vi "折叠行_symbols.vi"(8 "错误输入（无错误）":errorcluster, 11 "引用":refnum<k24>) -> (0 "错误输出":errorcluster, 3 "引用输出":refnum<k24>)   [LabVIEW 2018]
uses:
  ScintillaNET.dll
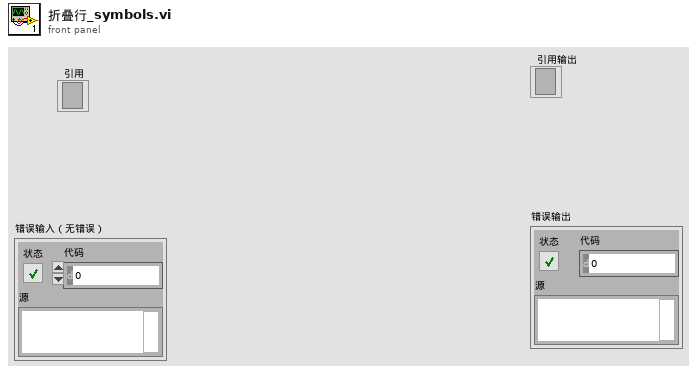
[diagram p1: front panel]
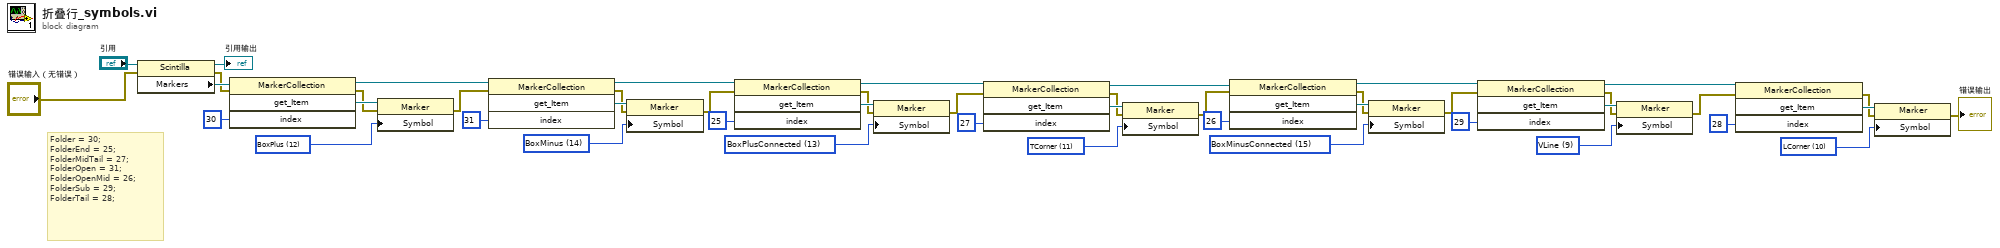
[diagram p0: block diagram]
diagram:
  w20 = 10 items=["Circle"=0, "RoundRect"=1, "Arrow"=2, "SmallRect"=3, "ShortArrow"=4, "Empty"=5, "ArrowDown"=6, "Minus"=7, "Plus"=8, "VLine"=9, "LCorner"=10, "TCorner"=11, "BoxPlus"=12, "BoxPlusConnected"=13, "BoxMinus"=14, "BoxMinusConnected"=15, "LCornerCurve"=16, "TCornerCurve"=17, "CirclePlus"=18, "CirclePlusConnected"=19, "CircleMinus"=20, "CircleMinusConnected"=21, "Background"=22, "DotDotDot"=23, "Arrows"=24, "FullRect"=26, "LeftRect"=27, "Available"=28, "Underline"=29, "RgbaImage"=30, "Bookmark"=31] ("Symbol")
  w22 = 9 items=["Circle"=0, "RoundRect"=1, "Arrow"=2, "SmallRect"=3, "ShortArrow"=4, "Empty"=5, "ArrowDown"=6, "Minus"=7, "Plus"=8, "VLine"=9, "LCorner"=10, "TCorner"=11, "BoxPlus"=12, "BoxPlusConnected"=13, "BoxMinus"=14, "BoxMinusConnected"=15, "LCornerCurve"=16, "TCornerCurve"=17, "CirclePlus"=18, "CirclePlusConnected"=19, "CircleMinus"=20, "CircleMinusConnected"=21, "Background"=22, "DotDotDot"=23, "Arrows"=24, "FullRect"=26, "LeftRect"=27, "Available"=28, "Underline"=29, "RgbaImage"=30, "Bookmark"=31] ("Symbol")
  w28 = 15 items=["Circle"=0, "RoundRect"=1, "Arrow"=2, "SmallRect"=3, "ShortArrow"=4, "Empty"=5, "ArrowDown"=6, "Minus"=7, "Plus"=8, "VLine"=9, "LCorner"=10, "TCorner"=11, "BoxPlus"=12, "BoxPlusConnected"=13, "BoxMinus"=14, "BoxMinusConnected"=15, "LCornerCurve"=16, "TCornerCurve"=17, "CirclePlus"=18, "CirclePlusConnected"=19, "CircleMinus"=20, "CircleMinusConnected"=21, "Background"=22, "DotDotDot"=23, "Arrows"=24, "FullRect"=26, "LeftRect"=27, "Available"=28, "Underline"=29, "RgbaImage"=30, "Bookmark"=31] ("Symbol")
  w30 = 11 items=["Circle"=0, "RoundRect"=1, "Arrow"=2, "SmallRect"=3, "ShortArrow"=4, "Empty"=5, "ArrowDown"=6, "Minus"=7, "Plus"=8, "VLine"=9, "LCorner"=10, "TCorner"=11, "BoxPlus"=12, "BoxPlusConnected"=13, "BoxMinus"=14, "BoxMinusConnected"=15, "LCornerCurve"=16, "TCornerCurve"=17, "CirclePlus"=18, "CirclePlusConnected"=19, "CircleMinus"=20, "CircleMinusConnected"=21, "Background"=22, "DotDotDot"=23, "Arrows"=24, "FullRect"=26, "LeftRect"=27, "Available"=28, "Underline"=29, "RgbaImage"=30, "Bookmark"=31] ("Symbol")
  w36 = 13 items=["Circle"=0, "RoundRect"=1, "Arrow"=2, "SmallRect"=3, "ShortArrow"=4, "Empty"=5, "ArrowDown"=6, "Minus"=7, "Plus"=8, "VLine"=9, "LCorner"=10, "TCorner"=11, "BoxPlus"=12, "BoxPlusConnected"=13, "BoxMinus"=14, "BoxMinusConnected"=15, "LCornerCurve"=16, "TCornerCurve"=17, "CirclePlus"=18, "CirclePlusConnected"=19, "CircleMinus"=20, "CircleMinusConnected"=21, "Background"=22, "DotDotDot"=23, "Arrows"=24, "FullRect"=26, "LeftRect"=27, "Available"=28, "Underline"=29, "RgbaImage"=30, "Bookmark"=31] ("Symbol")
  w37 = 14 items=["Circle"=0, "RoundRect"=1, "Arrow"=2, "SmallRect"=3, "ShortArrow"=4, "Empty"=5, "ArrowDown"=6, "Minus"=7, "Plus"=8, "VLine"=9, "LCorner"=10, "TCorner"=11, "BoxPlus"=12, "BoxPlusConnected"=13, "BoxMinus"=14, "BoxMinusConnected"=15, "LCornerCurve"=16, "TCornerCurve"=17, "CirclePlus"=18, "CirclePlusConnected"=19, "CircleMinus"=20, "CircleMinusConnected"=21, "Background"=22, "DotDotDot"=23, "Arrows"=24, "FullRect"=26, "LeftRect"=27, "Available"=28, "Underline"=29, "RgbaImage"=30, "Bookmark"=31] ("Symbol")
  w40 = 12 items=["Circle"=0, "RoundRect"=1, "Arrow"=2, "SmallRect"=3, "ShortArrow"=4, "Empty"=5, "ArrowDown"=6, "Minus"=7, "Plus"=8, "VLine"=9, "LCorner"=10, "TCorner"=11, "BoxPlus"=12, "BoxPlusConnected"=13, "BoxMinus"=14, "BoxMinusConnected"=15, "LCornerCurve"=16, "TCornerCurve"=17, "CirclePlus"=18, "CirclePlusConnected"=19, "CircleMinus"=20, "CircleMinusConnected"=21, "Background"=22, "DotDotDot"=23, "Arrows"=24, "FullRect"=26, "LeftRect"=27, "Available"=28, "Underline"=29, "RgbaImage"=30, "Bookmark"=31] ("Symbol")
  # "Folder = 30;\nFolderEnd = 25; \nFolderMidTail = 27;\nFolderOpen = 31;\nFolderOpenMid = 26;\nFolderSub = 29;\nFolderTail = 28;"
  n1 = property on="属性节点" class="Scintilla"(reference="引用", error in="错误输入（无错误）") -> (reference out=→"引用输出":refnum<k24>, error out=w16:errorcluster, "Markers"=w46:refnum<k24>)
  n2 = invoke class="MarkerCollection" method="get_Item"(reference=w46, error in=w16, "index"=30) -> (reference out=w43:refnum<k24>, error out=w15:errorcluster, "get_Item"=w41:refnum<k24>)  [unwired: 1 in, 1 out]
  n3 = property class="Marker"(reference=w41, error in=w15, "Symbol"=w40) -> (error out=w14:errorcluster)  [unwired: 1 out]
  n4 = invoke class="MarkerCollection" method="get_Item"(reference=w43, error in=w14, "index"=31) -> (reference out=w33:refnum<k24>, error out=w13:errorcluster, "get_Item"=w38:refnum<k24>)  [unwired: 1 in, 1 out]
  n5 = property class="Marker"(reference=w38, error in=w13, "Symbol"=w37) -> (error out=w12:errorcluster)  [unwired: 1 out]
  n6 = invoke class="MarkerCollection" method="get_Item"(reference=w33, error in=w12, "index"=25) -> (reference out=w29:refnum<k24>, error out=w11:errorcluster, "get_Item"=w35:refnum<k24>)  [unwired: 1 in, 1 out]
  n7 = property class="Marker"(reference=w35, error in=w11, "Symbol"=w36) -> (error out=w10:errorcluster)  [unwired: 1 out]
  n8 = invoke class="MarkerCollection" method="get_Item"(reference=w29, error in=w10, "index"=27) -> (reference out=w25:refnum<k24>, error out=w9:errorcluster, "get_Item"=w31:refnum<k24>)  [unwired: 1 in, 1 out]
  n9 = property class="Marker"(reference=w31, error in=w9, "Symbol"=w30) -> (error out=w8:errorcluster)  [unwired: 1 out]
  n10 = invoke class="MarkerCollection" method="get_Item"(reference=w25, error in=w8, "index"=26) -> (reference out=w21:refnum<k24>, error out=w7:errorcluster, "get_Item"=w27:refnum<k24>)  [unwired: 1 in, 1 out]
  n11 = property class="Marker"(reference=w27, error in=w7, "Symbol"=w28) -> (error out=w6:errorcluster)  [unwired: 1 out]
  n12 = invoke class="MarkerCollection" method="get_Item"(reference=w21, error in=w6, "index"=29) -> (reference out=w17:refnum<k24>, error out=w5:errorcluster, "get_Item"=w23:refnum<k24>)  [unwired: 1 in, 1 out]
  n13 = property class="Marker"(reference=w23, error in=w5, "Symbol"=w22) -> (error out=w4:errorcluster)  [unwired: 1 out]
  n14 = invoke class="MarkerCollection" method="get_Item"(reference=w17, error in=w4, "index"=28) -> (error out=w3:errorcluster, "get_Item"=w19:refnum<k24>)  [unwired: 1 in, 2 out]
  n15 = property class="Marker"(reference=w19, error in=w3, "Symbol"=w20) -> (error out=→"错误输出":errorcluster)  [unwired: 1 out]
